vi "Glimpse get new coefficients.vi"(0 "Coefficients":dbl[](array[numeric]) format="%0.2f", 1 "Alpha":dbl[][](array[numeric]) format="%0.2f", 9 "Beta":dbl[](array[numeric]) format="%0.2f", 11 "Fit this coeff?":bool[](array[boolean]), 12 "lamda":dbl format="%0.2e") -> (3 "New Coefficients":dbl[](array[numeric]) format="%0.2f", 14 "error":i32)   [LabVIEW 2016]
doc: "This subprogram is derived from a subprogram contained in the National Instruments LabView advanced analysis library. The original subprogram is copyright National Instruments."
uses:
  <resource>/lvanlys.dll
panel:
  # "(Modified from NI's \n\"Get New Coefficients\")"
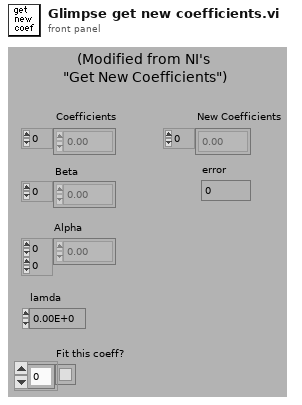
[diagram p1: front panel]
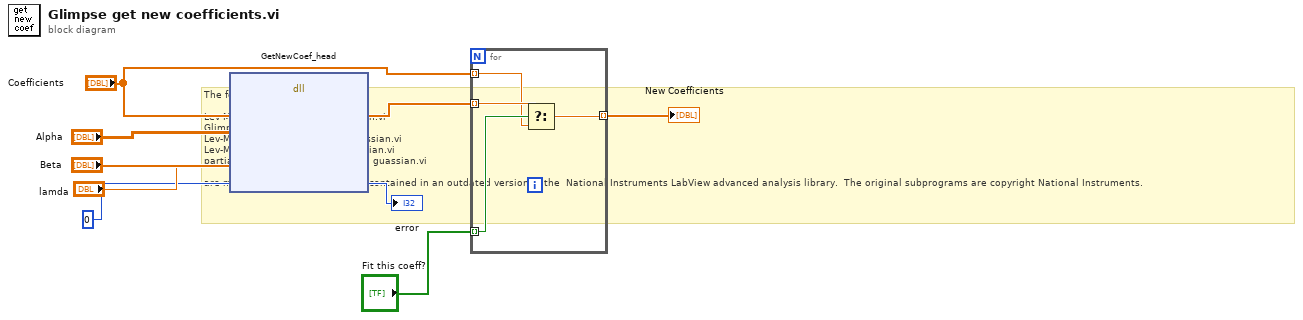
[diagram p0: block diagram]
diagram:
  # "The following subprograms:\n\nLev-Mar Fit to encoded 2D gaussian.vi\nGlimpse get new coefficients.vi\nLev-Mar abx with 2D encoded Gaussian.vi\nLev-Mar xx with 2D encoded Gaussian.vi\npartial derivative with 2D encoded guassian.vi\n\nare modifications of subprograms contained in an outdated version of the  National Instruments LabView advanced analysis library.  The original subprograms are copyright National Instruments."
  n1 = dll-call lib="C:/Program Files (x86)/National Instruments/LabVIEW 2016/resource/lvanlys.dll" fn="GetNewCoef_head"("coefH"="Coefficients", "alphaH"="Alpha", "betaH"="Beta", "lamda"="lamda", "err"=0) -> ("coefH"=w4:dbl[], "err"=→"error":i32)  [unwired: 6 in, 3 out]
  n2 = for {
    tunnel: w4 -> [w13] mode=indexing
    tunnel: "Fit this coeff?" -> [w11] mode=indexing
    tunnel: [w12] -> w2 mode=indexing
    tunnel: "Coefficients" -> [w10] mode=indexing
    n3 = Select(t=w13, s=w11, f=w10) -> (s? t:f=w12:dbl)
  }
  "New Coefficients" <- w2
